vi "Bank Tester.vi"(8 "entrée d'erreur (pas d'erreur)":errorcluster) -> (0 "sortie d'erreur":errorcluster)   [LabVIEW 2009]
uses:
  Account Info.ctl
  Stop.vi
panel:
  in  "Commande":T1
  in  "Montant à créditer":dbl
  in  "Montant à débiter":dbl
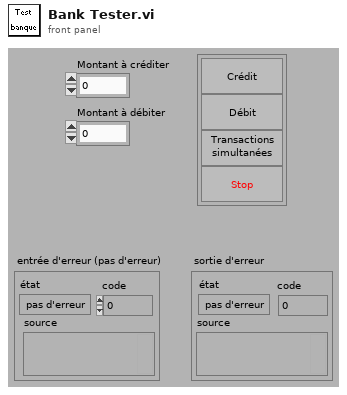
[diagram p1: front panel]
types:
  T1 = cluster{"Dépôt":bool, "Débit":bool, "Simultanés":bool, "Simultanés 2":bool}
  T2 = typedef "Account Info.ctl" = cluster{"Rendez-vous Banque":T3, "File d'attente des débits":refnum<queue>, "File d'attente des crédits":refnum<queue>}
  T3 = typedef "Rendezvous RefNum" = refnum<k1>
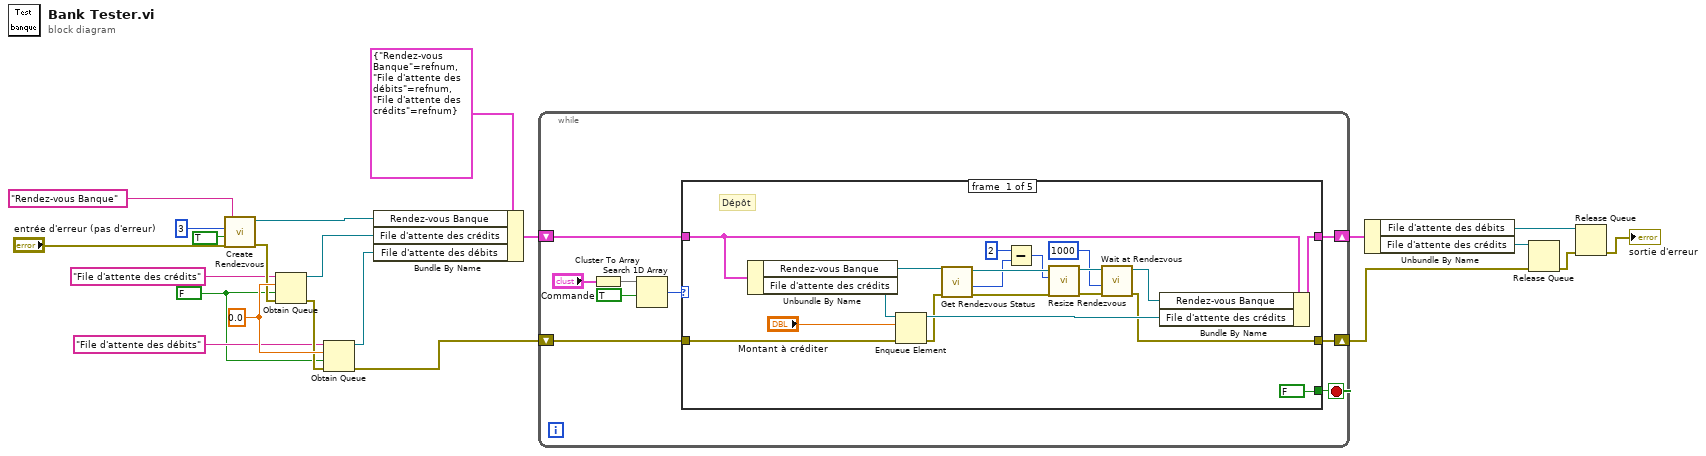
[diagram p0: block diagram]
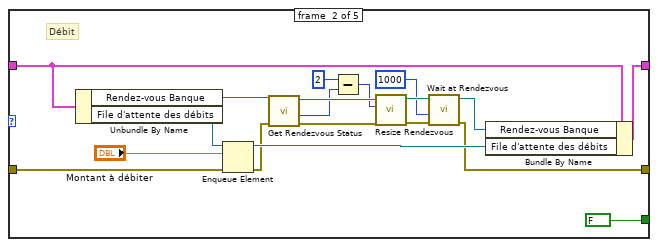
[diagram p2: hidden frame]
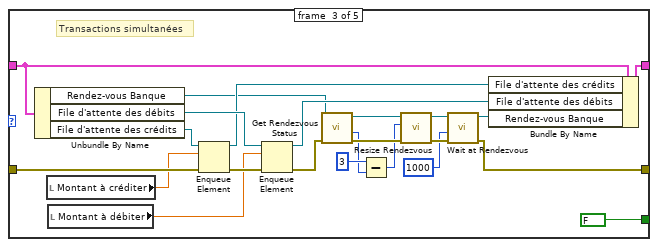
[diagram p3: hidden frame]
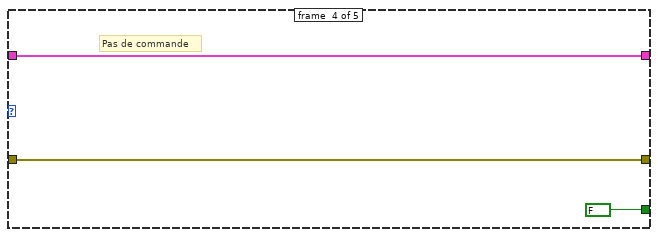
[diagram p4: hidden frame]
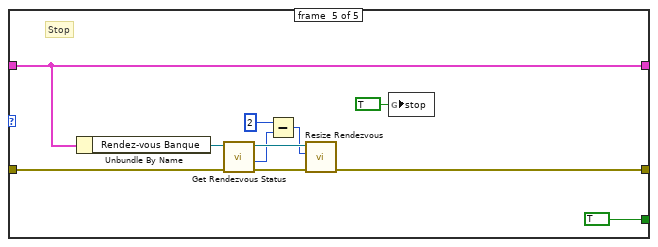
[diagram p5: hidden frame]
diagram:
  w1 = FALSE ("return existing (F)")
  w21 = 0.0
  n1 = call <vilib>:"Create Rendezvous.vi"("error in (no error)"="entrée d'erreur (pas d'erreur)", "return existing (F)"=TRUE, "size (2)"=3, "name (unnamed)"="Rendez-vous Banque") -> ("error out"=w20:errorcluster, "rendezvous"=w22:T3)  [unwired: 2 out]
  n2 = Obtain Queue ("Obtenir une file d'attente")(name (unnamed)="File d'attente des crédits", element data type=w21, create if not found? (T)=w1, error in (no error)=w20) -> (queue out=w18:refnum<queue>, error out=w19:errorcluster)  [unwired: 1 in, 1 out]
  n3 = Obtain Queue ("Obtenir une file d'attente")(name (unnamed)="File d'attente des débits", element data type=w21, create if not found? (T)=w1, error in (no error)=w19) -> (queue out=w17:refnum<queue>, error out=w9:errorcluster)  [unwired: 1 in, 1 out]
  n4 = Bundle By Name ("Assembler par nom")(cluster=T2 {"Rendez-vous Banque"=refnum, "File d'attente des débits"=refnum, "File d'attente des crédits"=refnum} ("Account info"), "Rendez-vous Banque"=w22, "File d'attente des crédits"=w18, "File d'attente des débits"=w17) -> (w11:T2)
  n5 = while "Boucle While" {
    shift-right: [w25] -> w4
    shift-left: w9 -> [w24]
    shift-right: [w26] -> w8
    shift-left: w11 -> [w28]
    stop <- w23 stop-if-true
    n6 = Cluster To Array ("Cluster en tableau")(cluster="Commande") -> (array=w30:bool[])
    n7 = Search 1D Array ("Rechercher dans un tableau 1D")(1D array=w30, element=TRUE) -> (index of element=w29:i32)  [unwired: 1 out]
    n8 = case "Structure Condition" shown="0" w29 {
      tunnel: w28 -> [w32 w51 w88 w95 w104]
      tunnel: w24 -> [w48 w68 w85 w94 w100]
      tunnel: [w43 w63 w89 w95 w104] -> w26
      tunnel: [w42 w62 w87 w94 w96] -> w25
      tunnel: [FALSE FALSE FALSE FALSE TRUE] -> w23
      frame #0 {
        # "Dépôt"
        n9 = Unbundle By Name(w32) -> ("Rendez-vous Banque"=w37:T3, "File d'attente des crédits"=w50:refnum<queue>)
        n10 = Enqueue Element(queue=w50, element="Montant à créditer", error in (no error)=w48) -> (queue out=w44:refnum<queue>, error out=w39:errorcluster)  [unwired: 2 out]
        n11 = call <vilib>:"Get Rendezvous Status.vi"("error in (no error)"=w39, "rendezvous"=w37) -> ("error out"=w38:errorcluster, "size"=w34:i32, "rendezvous out"=w36:T3)  [unwired: 7 out]
        n12 = Subtract(x=2 ("size change (0)"), y=w34) -> (x-y=w33:i32)
        n13 = call <vilib>:"Resize Rendezvous.vi"("error in (no error)"=w38, "size change (0)"=w33, "rendezvous"=w36) -> ("error out"=w47:errorcluster, "rendezvous out"=w46:T3)  [unwired: 3 out]
        n14 = call <vilib>:"Wait at Rendezvous.vi"("error in (no error)"=w47, "ms timeout (-1)"=1000, "rendezvous"=w46) -> ("error out"=w42:errorcluster, "rendezvous out"=w45:T3)  [unwired: 3 out]
        n15 = Bundle By Name(cluster=w32, "Rendez-vous Banque"=w45, "File d'attente des crédits"=w44) -> (w43:T2)
      }
      frame #1 {
        # "Débit"
        n16 = Unbundle By Name(w51) -> ("Rendez-vous Banque"=w57:T3, "File d'attente des débits"=w69:refnum<queue>)
        n17 = Enqueue Element(queue=w69, element="Montant à débiter", error in (no error)=w68) -> (queue out=w64:refnum<queue>, error out=w59:errorcluster)  [unwired: 2 out]
        n18 = call <vilib>:"Get Rendezvous Status.vi"("error in (no error)"=w59, "rendezvous"=w57) -> ("error out"=w58:errorcluster, "size"=w54:i32, "rendezvous out"=w56:T3)  [unwired: 7 out]
        n19 = Subtract(x=2 ("size change (0)"), y=w54) -> (x-y=w53:i32)
        n20 = call <vilib>:"Resize Rendezvous.vi"("error in (no error)"=w58, "size change (0)"=w53, "rendezvous"=w56) -> ("error out"=w67:errorcluster, "rendezvous out"=w66:T3)  [unwired: 3 out]
        n21 = call <vilib>:"Wait at Rendezvous.vi"("error in (no error)"=w67, "ms timeout (-1)"=1000, "rendezvous"=w66) -> ("error out"=w62:errorcluster, "rendezvous out"=w65:T3)  [unwired: 3 out]
        n22 = Bundle By Name(cluster=w51, "Rendez-vous Banque"=w65, "File d'attente des débits"=w64) -> (w63:T2)
      }
      frame #2 {
        # "Transactions simultanées"
        n23 = Unbundle By Name(w88) -> ("Rendez-vous Banque"=w76:T3, "File d'attente des débits"=w92:refnum<queue>, "File d'attente des crédits"=w86:refnum<queue>)
        n24 = local read "Montant à créditer"() -> (w80:dbl)
        n25 = local read "Montant à débiter"() -> (w79:dbl)
        n26 = Enqueue Element(queue=w86, element=w80, error in (no error)=w85) -> (queue out=w83:refnum<queue>, error out=w84:errorcluster)  [unwired: 2 out]
        n27 = Enqueue Element(queue=w92, element=w79, error in (no error)=w84) -> (queue out=w81:refnum<queue>, error out=w75:errorcluster)  [unwired: 2 out]
        n28 = call <vilib>:"Get Rendezvous Status.vi"("error in (no error)"=w75, "rendezvous"=w76) -> ("error out"=w74:errorcluster, "size"=w71:i32, "rendezvous out"=w73:T3)  [unwired: 7 out]
        n29 = Subtract(x=3 ("size change (0)"), y=w71) -> (x-y=w70:i32)
        n30 = call <vilib>:"Resize Rendezvous.vi"("error in (no error)"=w74, "size change (0)"=w70, "rendezvous"=w73) -> ("error out"=w91:errorcluster, "rendezvous out"=w90:T3)  [unwired: 3 out]
        n31 = call <vilib>:"Wait at Rendezvous.vi"("error in (no error)"=w91, "ms timeout (-1)"=1000, "rendezvous"=w90) -> ("error out"=w87:errorcluster, "rendezvous out"=w82:T3)  [unwired: 3 out]
        n32 = Bundle By Name(cluster=w88, "File d'attente des crédits"=w83, "File d'attente des débits"=w81, "Rendez-vous Banque"=w82) -> (w89:T2)
      }
      frame #3 {
        # "Pas de commande"
      }
      frame #4 {
        # "Stop"
        n33 = Unbundle By Name(w104) -> ("Rendez-vous Banque"=w101:T3)
        n34 = call <vilib>:"Get Rendezvous Status.vi"("error in (no error)"=w100, "rendezvous"=w101) -> ("error out"=w103:errorcluster, "size"=w99:i32, "rendezvous out"=w102:T3)  [unwired: 7 out]
        n35 = Subtract(x=2, y=w99) -> (x-y=w97:i32)
        n36 = call <vilib>:"Resize Rendezvous.vi"("error in (no error)"=w103, "size change (0)"=w97, "rendezvous"=w102) -> ("error out"=w96:errorcluster)  [unwired: 4 out]
        n37 = global write "Stop.vi" "stop"(TRUE ("stop")) -> ()
      }
    }
  }
  n38 = Unbundle By Name ("Désassembler par nom")(w8) -> ("File d'attente des débits"=w6:refnum<queue>, "File d'attente des crédits"=w7:refnum<queue>)
  n39 = Release Queue ("Libérer une file d'attente")(queue=w7, error in (no error)=w4) -> (error out=w5:errorcluster)  [unwired: 3 out]
  n40 = Release Queue ("Libérer une file d'attente")(queue=w6, error in (no error)=w5) -> (error out=→"sortie d'erreur":errorcluster)  [unwired: 3 out]
